vi "Dispose.vi"(8 "error in":errorcluster, 10 "Dispose All":bool, 11 "Image Reference In":T1) -> (0 "error out":errorcluster)   [LabVIEW 2020, in "OpenLvVision_Image.lvlib" / "Management.lvlib"]
doc: "Disposes of a previously generated image. This method releases the memory and resources associated with a specific image object, often identified internally (e.g., as a \"dellacote image\"), that is no longer required."
uses:
  Management.lvlib
  TypeDef/Image.ctl
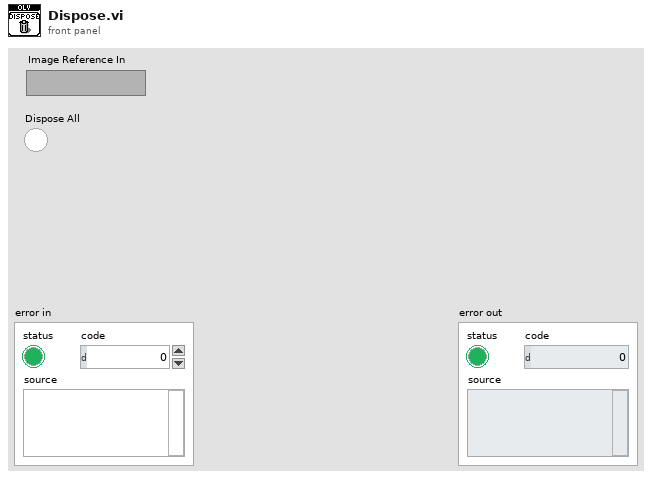
[diagram p1: front panel]
types:
  T1 = typedef "OpenLvVision_Image.lvlib/Management.lvlib/Image.ctl" = refnum<image>
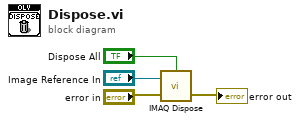
[diagram p0: block diagram]
diagram:
  n1 = call "IMAQ Dispose"("All Images? (No)"="Dispose All", "Image"="Image Reference In", "error in (no error)"="error in") -> ("error out"=→"error out":errorcluster)  [unwired: 3 in]
